vi "Read From JSON Data.vi"(11 "Mock JSON Serializable in":refnum<class "Mock JSON Serializable.lvclass">) -> (2 "From JSON Data":T1, 3 "Mock JSON Serializable out":refnum<class "Mock JSON Serializable.lvclass">)   [LabVIEW 2017, in "JSON Serializable Serializer Tests.lvlib" / "Mock JSON Serializable.lvclass"]
uses:
  Mock JSON Serializable.lvclass
  <vilib>/JDP Science/JSONtext/LVClass Serializer/JSONtext LVClass Serializer.lvclass
  Mock JSON Serializable.lvclass/Mock JSON Serializable.ctl
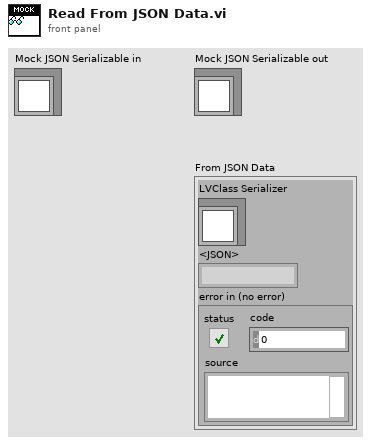
[diagram p1: front panel]
types:
  T1 = cluster{"LVClass Serializer":refnum<class "JSONtext LVClass Serializer.lvclass">, "<JSON>":string, "error in (no error)":errorcluster}
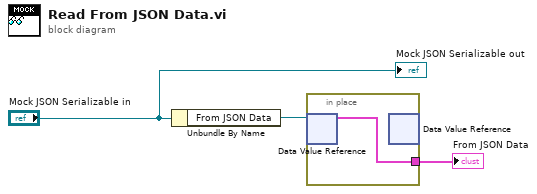
[diagram p0: block diagram]
diagram:
  n1 = Unbundle By Name("Mock JSON Serializable in") -> ("From JSON Data"=w2:refnum<data-value>)
  n2 = in-place {
    in-place-border: [w4] -> w1
    n3 = in-place-dvr #1(w2) -> (w4:T1)  [unwired: 1 out]
    n4 = in-place-dvr #1() -> ()  [unwired: 1 in, 2 out]
  }
  "From JSON Data" <- w1
  "Mock JSON Serializable out" <- "Mock JSON Serializable in"
